vi "clearpath_parse_platform_name.vi"(0 "ClearpathComm":T1) -> (1 "Data Valid?":bool=TRUE, 2 "Platform Name":string)   [LabVIEW 2010, in "clearpath_interface.lvlib"]
doc: "Parses platform name as returned by platform. (Message type 0x8002)"
uses:
  clearpath_interface.lvlib
  cwrap_cRIO.dll
panel:
  # "Platform Name"
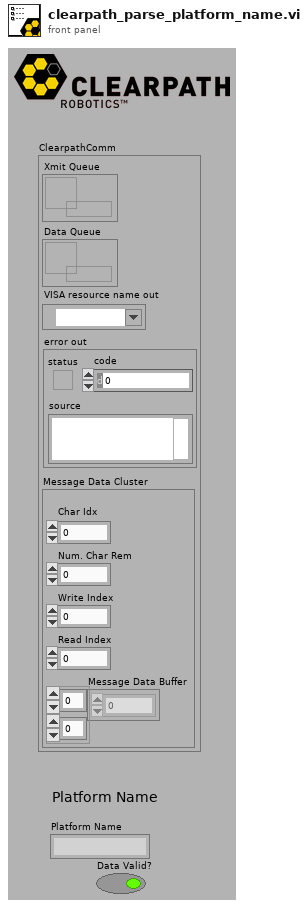
[diagram p1: front panel]
types:
  T1 = cluster{"Xmit Queue":refnum<queue>, "Data Queue":refnum<queue>, "VISA resource name out":refnum<visa-resource-name>, "error out":errorcluster, "Message Data Cluster":cluster{"\nChar Idx":u8, "Num. Char Rem":u8, "Write Index":u8, "Read Index":u8, "Message Data Buffer":u8[][]}}
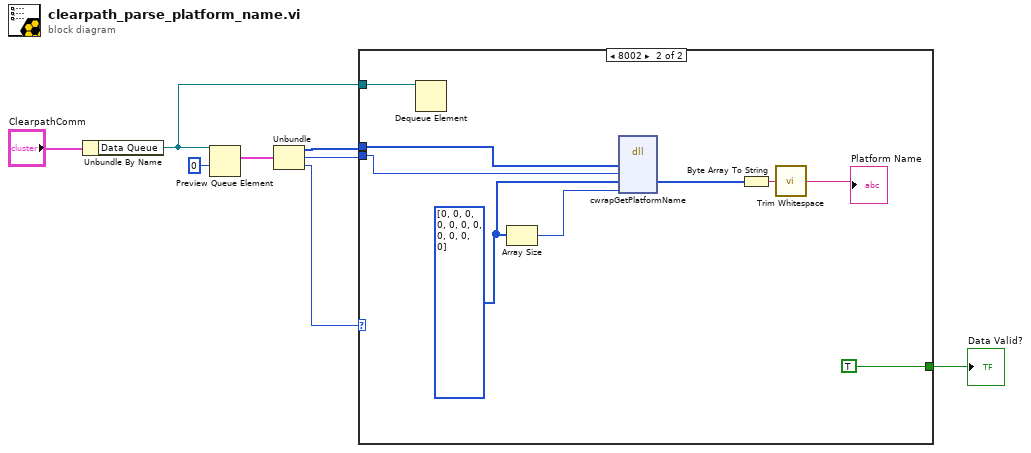
[diagram p0: block diagram]
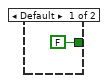
[diagram p2: hidden frame]
diagram:
  n1 = Unbundle By Name("ClearpathComm") -> ("Data Queue"=w1:refnum<queue>)
  n2 = Preview Queue Element(queue=w1, timeout in ms (-1)=0) -> (element=w6:cluster{u8[], "Length":i32, "Type":i32})  [unwired: 1 in, 3 out]
  n3 = Unbundle(w6) -> (w3:u8[], "Length"=w4:i32, "Type"=w5:i32)
  n4 = case shown="8002" w5 {
    tunnel: w4 -> [_ w12]
    tunnel: w3 -> [_ w13]
    tunnel: [FALSE TRUE] -> w2
    tunnel: w1 -> [_ w10]
    frame Default {
    }
    frame 32770 {
      w18 = i32[] [0, 0, 0, 0, 0, 0, 0, 0, 0, 0, 0] ("Array")
      n5 = Dequeue Element(queue=w10) -> ()  [unwired: 2 in, 4 out]
      n6 = Array Size(array=w18) -> (size(s)=w17:i32)
      n7 = dll-call lib="cwrap_cRIO.*" fn="cwrapGetPlatformName"("packet"=w13, "len"=w12, "name"=w18, "name_len"=w17) -> ("name"=w16:i8[])  [unwired: 7 in, 2 out]
      n8 = Byte Array To String(unsigned byte array=w16) -> (string=w15:string)
      n9 = call <vilib>:"Trim Whitespace.vi"("string"=w15) -> ("trimmed string"=→"Platform Name":string)  [unwired: 1 in]
    }
  }
  "Data Valid?" <- w2
